vi "Set Payload.vi"(10 "Payload":u8[](array[numeric]), 11 "CAN Frame in":refnum<class "CAN Frame.lvclass">) -> (3 "CAN Frame out":refnum<class "CAN Frame.lvclass">)   [LabVIEW 2023, in "CAN Frame.lvclass"]
uses:
  CAN Frame.lvclass
  CAN Frame.lvclass/CAN Frame.ctl
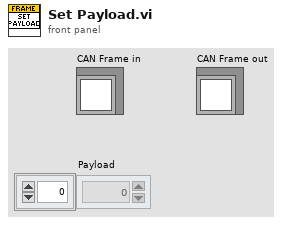
[diagram p1: front panel]
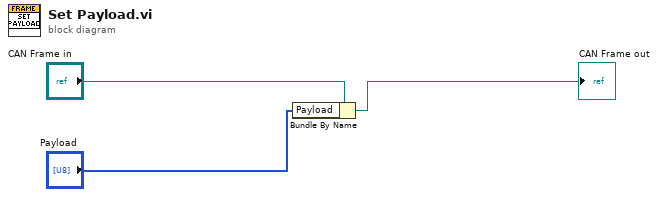
[diagram p0: block diagram]
diagram:
  n1 = Bundle By Name(cluster="CAN Frame in", "Payload"="Payload") -> (→"CAN Frame out":refnum<class "CAN Frame.lvclass">)
